vi "Advanced data viewer.vi"() -> ()   [LabVIEW 2016]
uses:
  <vilib>/Utility/miscctls.llb/LV3DPointTypeDef.ctl
  Typedef/Advancer viewer - States.ctl
  <vilib>/picture/3D Picture Control/Object/Create Object (name).vi
  <vilib>/picture/3D Picture Control/NI_3D Picture Control.lvlib
panel:
  out "Intensity Graph":sgl[][](graph)
  in  "Clear plot":bool
  out "Strain 1-8 Zoom":T1(graph)
  out "3D Picture":refnum<vi>(3d-picture)
  out "Strain 1-8":T1(graph)
  # "Yaw - Pitch - Roll - 3D"
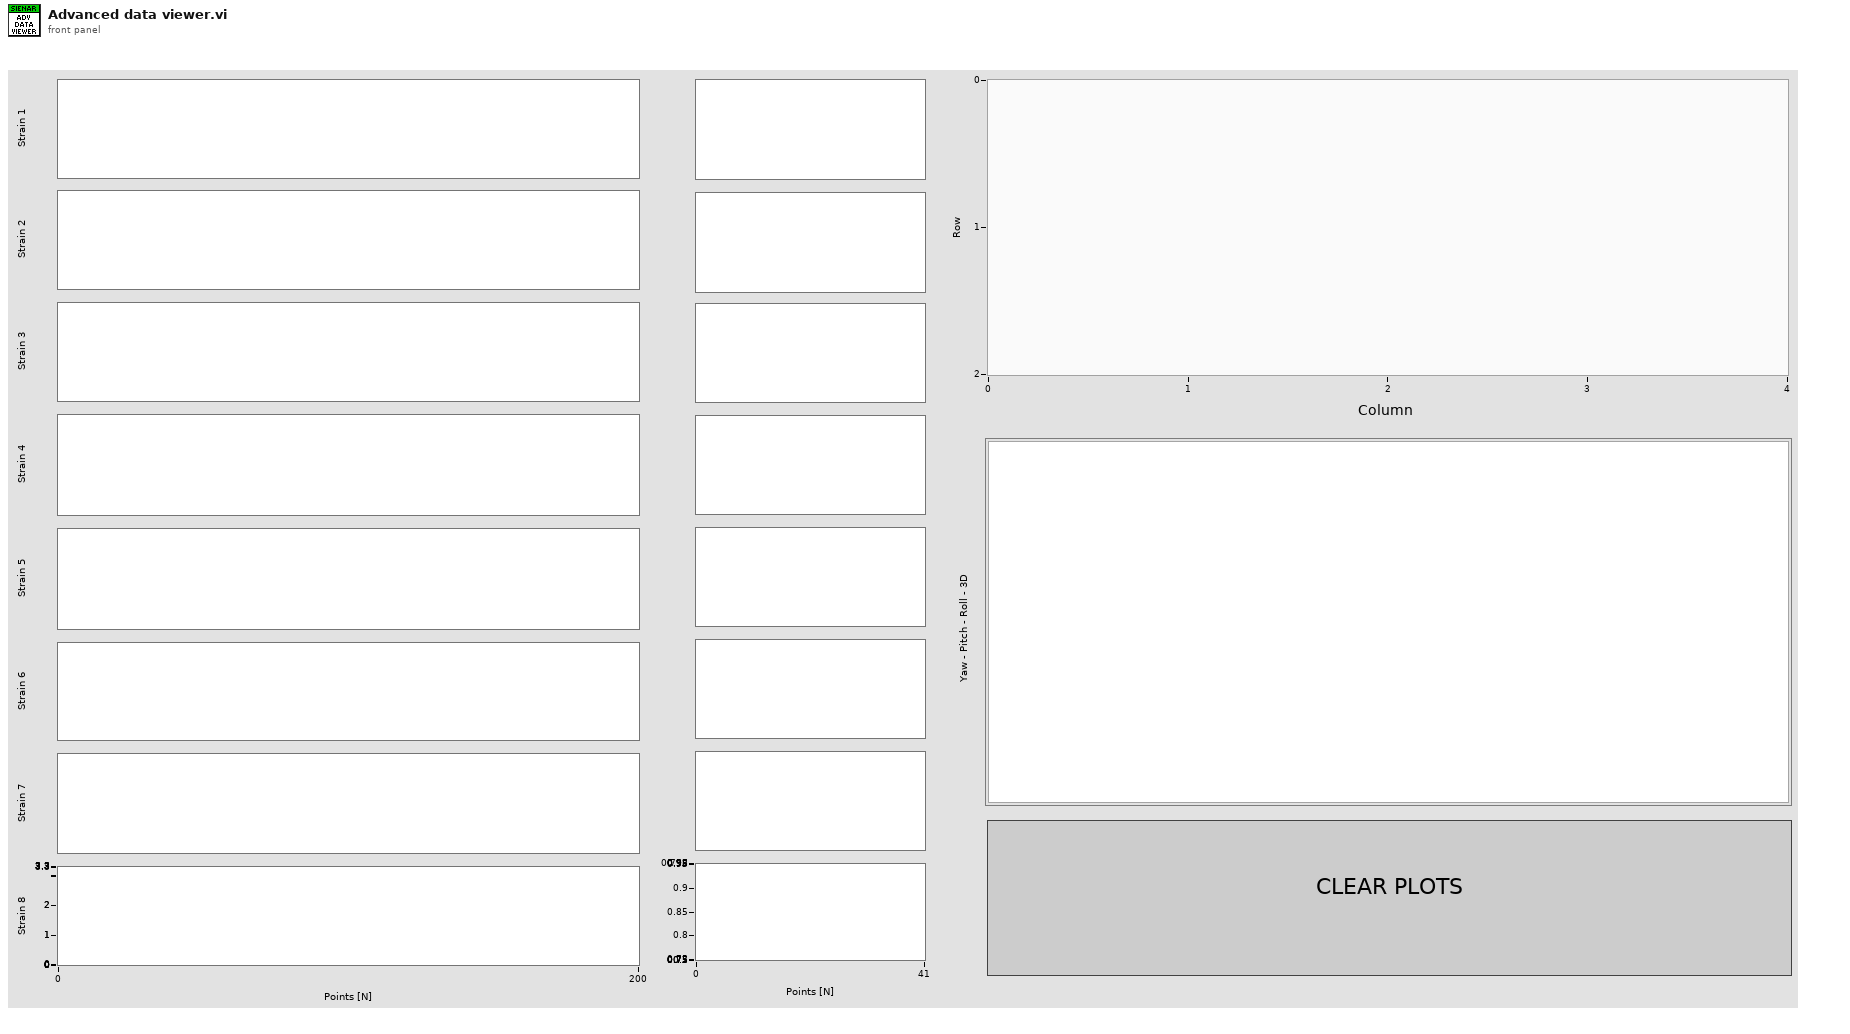
[diagram p1: front panel]
types:
  T1 = cluster{"Strain sensor 1":sgl, "Strain sensor 2":sgl, "Strain sensor 3":sgl, "Strain sensor 4":sgl, "Strain sensor 5":sgl, "Strain sensor 6":sgl, "Strain sensor 7":sgl, "Strain sensor 8":sgl}
  T2 = cluster{"Strain data":cluster{"Strain sensor 1":sgl, "Strain sensor 2":sgl, "Strain sensor 3":sgl, "Strain sensor 4":sgl, "Strain sensor 5":sgl, "Strain sensor 6":sgl, "Strain sensor 7":sgl, "Strain sensor 8":sgl}, "YPR data":cluster{"Yaw":sgl, "Pitch":sgl, "Roll":sgl}}
  T3 = typedef "Advancer viewer - States.ctl" = enum16{"Run data", "Exit"}
  T4 = typedef "LV3DPointTypeDef.ctl" = cluster{"X":sgl, "Y":sgl, "Z":sgl}
  T5 = cluster{"[0]":dbl, "[1]":dbl, "[2]":dbl, "[3]":dbl}[]
  T6 = cluster{"[0]":dbl, "[1]":dbl, "[2]":dbl, "[3]":dbl, "[4]":dbl, "[5]":dbl, "[6]":dbl, "[7]":dbl}[]
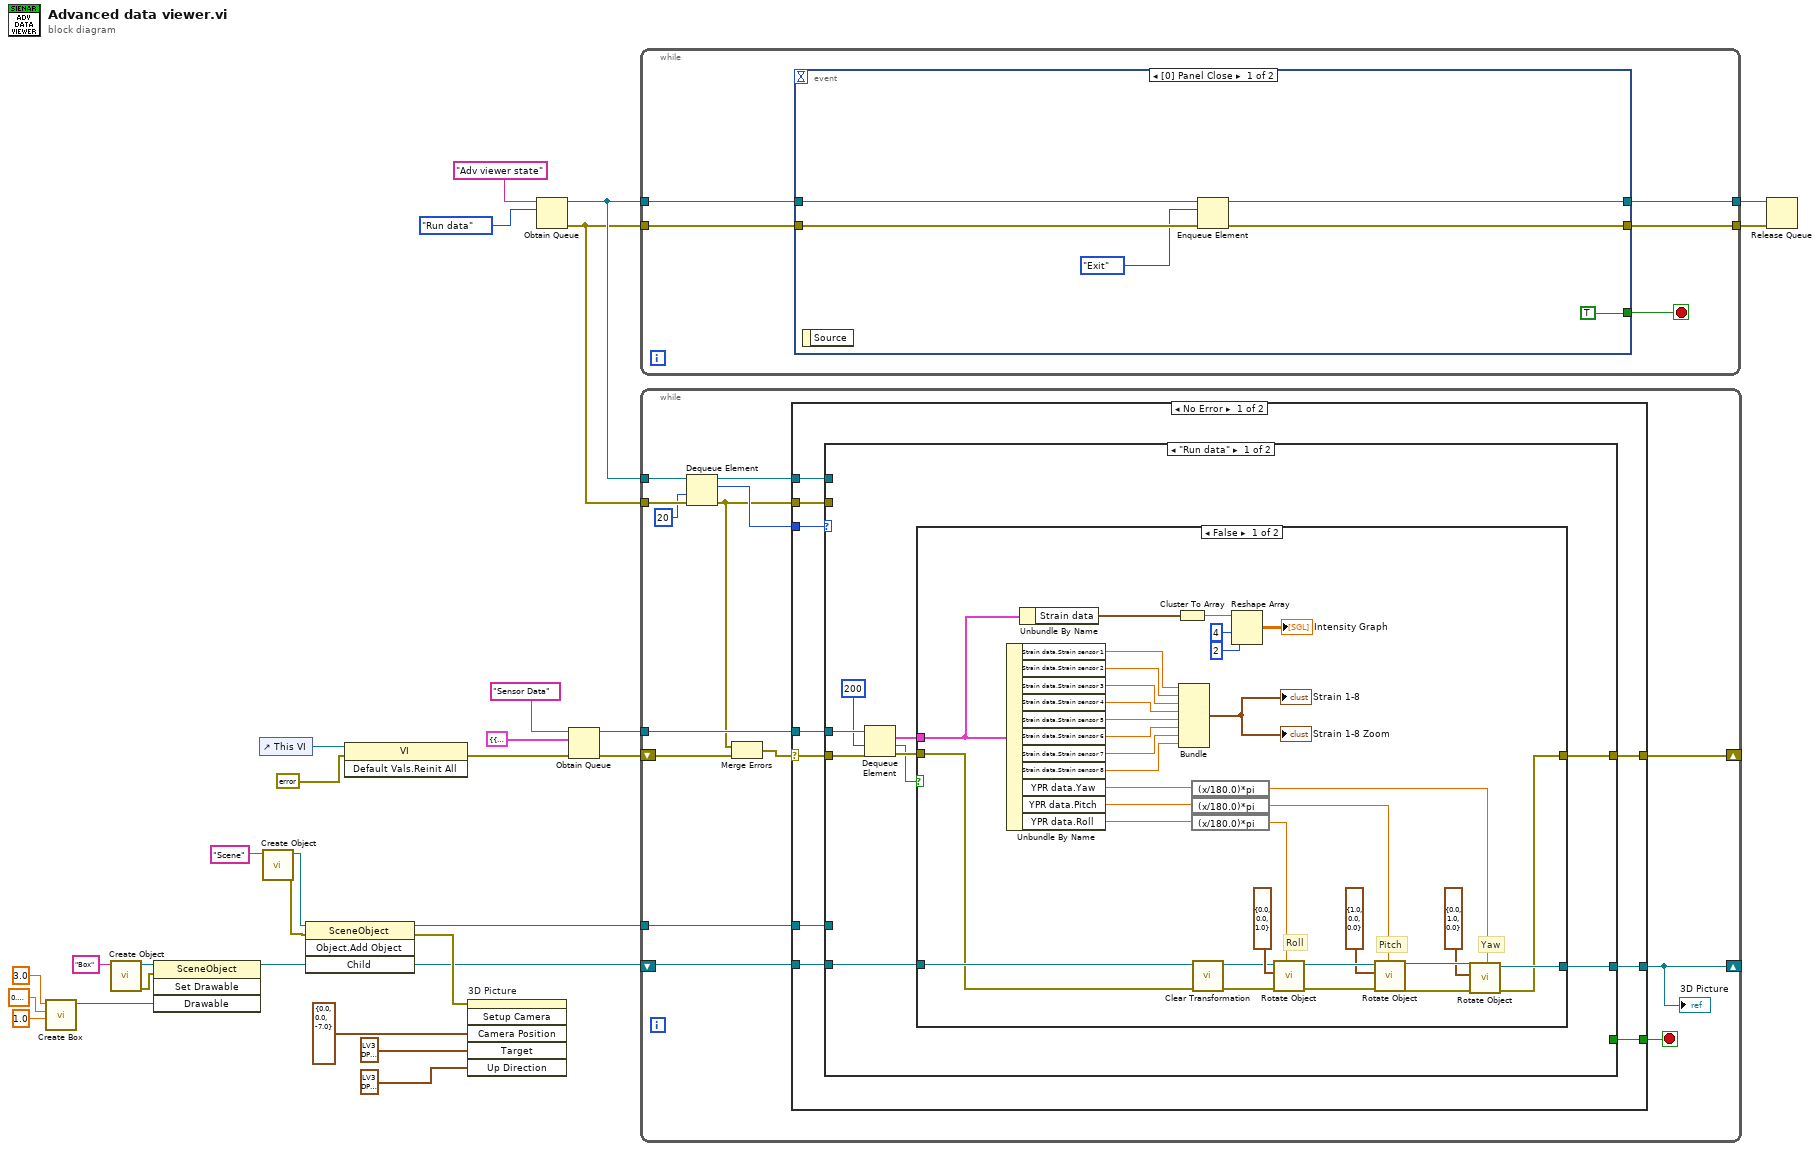
[diagram p0: block diagram]
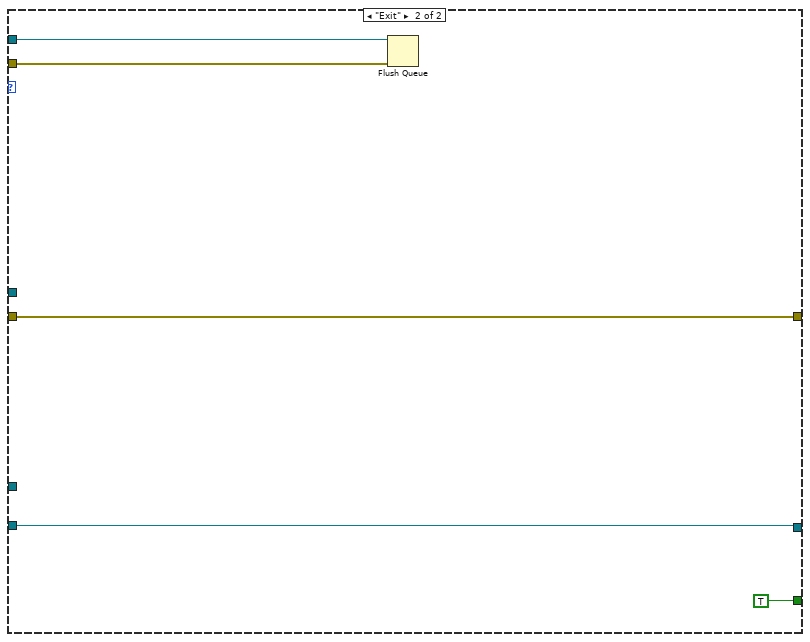
[diagram p3: hidden frame]
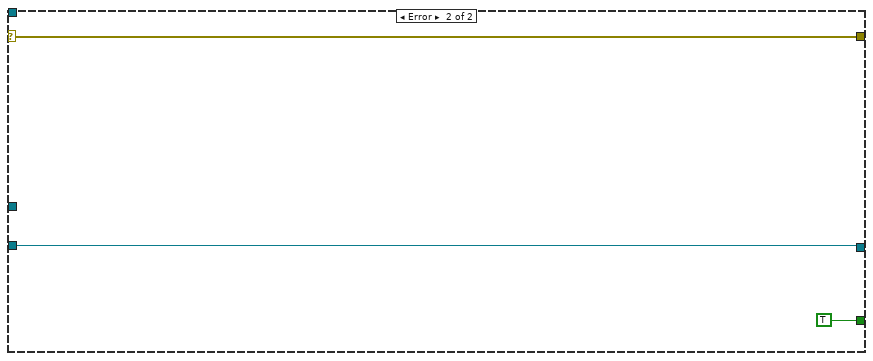
[diagram p4: hidden frame]
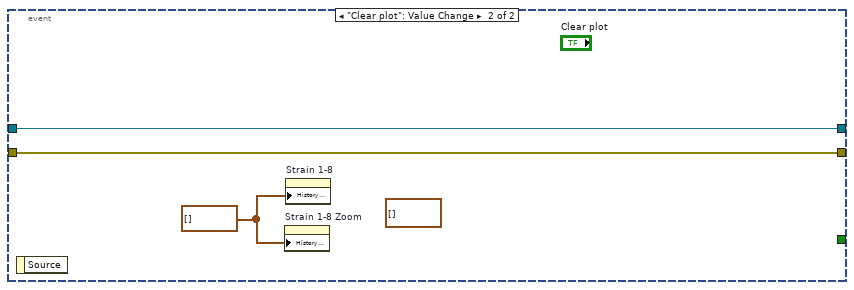
[diagram p5: hidden frame]
diagram:
  n1 = call <vilib>:"Create Box.vi"("Length Z"=sgl 1.0, "Length Y"=sgl 0.2, "Length X"=sgl 3.0) -> ("New Box Refnum"=w25:refnum<vi>)  [unwired: 7 in, 1 out]
  n2 = call-poly <vilib>:"Create Object.vi"("Name"="Box") -> ("error out"=w24:errorcluster, "Scene:New Object"=w23:refnum<vi>)  [unwired: 9 in]
  n3 = invoke class="SceneObject" method="Set Drawable"(reference=w23, error in=w24, "Drawable"=w25) -> (reference out=w29:refnum<vi>)  [unwired: 1 in, 3 out]
  n4 = control-ref of="This VI"() -> (w30:refnum<vi>)
  n5 = call-poly <vilib>:"Create Object.vi"("Name"="Scene") -> ("error out"=w28:errorcluster, "Scene:New Object"=w27:refnum<vi>)  [unwired: 9 in]
  n6 = invoke class="SceneObject" method="Object.Add Object"(reference=w27, error in=w28, "Child"=w29) -> (reference out=w5:refnum<vi>, error out=w15:errorcluster, "Child"=w6:refnum<vi>)  [unwired: 1 in, 1 out]
  n7 = invoke class="VI" method="Default Vals.Reinit All"(reference=w30, error in=errorcluster {"status"=FALSE, "code"=0, "source"=""} ("Error In")) -> (error out=w13:errorcluster)  [unwired: 1 in, 2 out]
  n8 = invoke on="3D Picture" class="SceneGraphDisp (strict)" method="Setup Camera"(error in=w15, "Camera Position"=T4 {"X"=0.0, "Y"=0.0, "Z"=-7.0}, "Target"=T4 {"X"=0.0, "Y"=0.0, "Z"=0.0}, "Up Direction"=T4 {"X"=0.0, "Y"=1.0, "Z"=0.0}) -> ()  [unwired: 2 in, 6 out]
  n9 = Obtain Queue(name (unnamed)="Adv viewer state", element data type=Advancer_viewer_-_States."Run data") -> (queue out=w11:refnum<queue>, error out=w10:errorcluster)  [unwired: 3 in, 1 out]
  n10 = Obtain Queue(name (unnamed)="Sensor Data", element data type=T2 {"Strain data"={"Strain sensor 1"=0.0, "Strain sensor 2"=0.0, "Strain sensor 3"=0.0, "Strain sensor 4"=0.0, "Strain sensor 5"=0.0, "Strain sensor 6"=0.0, "Strain sensor 7"=0.0, "Strain sensor 8"=0.0}, "YPR data"={"Yaw"=0.0, "Pitch"=0.0, "Roll"=0.0}} ("Wristband data"), error in (no error)=w13) -> (queue out=w8:refnum<queue>, error out=w7:errorcluster)  [unwired: 2 in, 1 out]
  n11 = while {
    tunnel: w11 -> [w34]
    tunnel: w10 -> [w33]
    tunnel: [w32] -> w3
    tunnel: [w31] -> w2
    stop <- w35 stop-if-true
    n12 = event shown="[0] Panel Close" {
      selector: _ -> [_ _]
      dyn-events: _ -> [_ _]
      timeout: _ -> [_ _]
      tunnel: [TRUE _] -> w35
      tunnel: w34 -> [w40 w42]
      tunnel: w33 -> [w39 w43]
      tunnel: [w38 w42] -> w32
      tunnel: [w37 w43] -> w31
      event Panel Close {
        n13 = event-data() -> ()  [unwired: 1 in, 1 out]
        n14 = Enqueue Element(queue=w40, element=Advancer_viewer_-_States."Exit", error in (no error)=w39) -> (queue out=w38:refnum<queue>, error out=w37:errorcluster)  [unwired: 1 in, 1 out]
      }
      event "Clear plot": Value Change {
        (unwired) T5 [] ("History Data")
        w44 = T6 [] ("History Data")
        n15 = event-data() -> ()  [unwired: 1 in, 1 out]
        n16 = property on="Strain 1-8 Zoom" class="WFChart (strict)"("History Data"=w44) -> ()  [unwired: 2 in, 2 out]
        n17 = property on="Strain 1-8" class="WFChart (strict)"("History Data"=w44) -> ()  [unwired: 2 in, 2 out]
      }
    }
  }
  n18 = while {
    tunnel: w11 -> [w58]
    tunnel: w10 -> [w57]
    tunnel: w8 -> [w55]
    tunnel: w5 -> [w53]
    shift-right: [w49] -> _
    shift-left: w6 -> [w54]
    shift-right: [w45] -> _
    shift-left: w7 -> [w48]
    stop <- w50 stop-if-true
    n19 = Dequeue Element(queue=w58, timeout in ms (-1)=20, error in (no error)=w57) -> (queue out=w52:refnum<queue>, element=w56:T3, error out=w46:errorcluster)  [unwired: 1 out]
    n20 = Merge Errors(w46, w48) -> (w47:errorcluster)
    n21 = case shown="No Error" w47 {
      selector: w47 -> [w60 w119]
      tunnel: w56 -> [w68 _]
      tunnel: w55 -> [w67 _]
      tunnel: w54 -> [w66 w120]
      tunnel: w53 -> [w65 _]
      tunnel: w52 -> [w64 _]
      tunnel: w46 -> [w63 _]
      tunnel: [w62 TRUE] -> w50
      tunnel: [w61 w120] -> w49
      tunnel: [w59 w119] -> w45
      frame No Error {
        n22 = case shown="\"Run data\"" w68 {
          tunnel: w67 -> [w77 _]
          tunnel: w60 -> [w76 w114]
          tunnel: w66 -> [w75 w115]
          tunnel: w65 -> [_ _]
          tunnel: w64 -> [_ w118]
          tunnel: w63 -> [_ w117]
          tunnel: [_ TRUE] -> w62
          tunnel: [w73 w115] -> w61
          tunnel: [w71 w114] -> w59
          frame "Run data" {
            n23 = Dequeue Element(queue=w77, timeout in ms (-1)=200, error in (no error)=w76) -> (element=w72:T2, timed out?=w70:bool, error out=w74:errorcluster)  [unwired: 1 out]
            n24 = case shown="False" w70 {
              tunnel: w75 -> [w100 w112]
              tunnel: w74 -> [w90 w113]
              tunnel: [w86 w112] -> w73
              tunnel: w72 -> [w85 _]
              tunnel: [w78 w113] -> w71
              frame False {
                # "Yaw"
                # "Pitch"
                # "Roll"
                n25 = Unbundle By Name(w85) -> ("Strain data.Strain sensor 1"=w108:sgl, "Strain data.Strain sensor 2"=w107:sgl, "Strain data.Strain sensor 3"=w106:sgl, "Strain data.Strain sensor 4"=w105:sgl, "Strain data.Strain sensor 5"=w104:sgl, "Strain data.Strain sensor 6"=w103:sgl, "Strain data.Strain sensor 7"=w102:sgl, "Strain data.Strain sensor 8"=w101:sgl, "YPR data.Yaw"=w81:sgl, "YPR data.Pitch"=w80:sgl, "YPR data.Roll"=w79:sgl)
                n26 = Unbundle By Name(w85) -> ("Strain data"=w84:T1)
                n27 = Cluster To Array(cluster=w84) -> (array=w109:sgl[])
                n28 = Bundle("Strain sensor 1"=w108, "Strain sensor 2"=w107, "Strain sensor 3"=w106, "Strain sensor 4"=w105, "Strain sensor 5"=w104, "Strain sensor 6"=w103, "Strain sensor 7"=w102, "Strain sensor 8"=w101) -> (→"Strain 1-8" →"Strain 1-8 Zoom":T1)  [unwired: 1 in]
                n29 = expression code="(x/180.0)*pi" ("degrees to radians")(w81) -> (w87:sgl)
                n30 = expression code="(x/180.0)*pi" ("degrees to radians")(w80) -> (w88:sgl)
                n31 = expression code="(x/180.0)*pi" ("degrees to radians")(w79) -> (w89:sgl)
                n32 = call <vilib>:"Clear Transformation.vi"("error in (no error)"=w90, "Object Refnum In"=w100) -> ("error out"=w91:errorcluster, "Object Refnum Out"=w92:refnum<vi>)  [unwired: 8 in]
                n33 = Reshape Array(w109, 4 ("dimension size"), 2 ("dimension size")) -> (→"Intensity Graph":sgl[][])
                n34 = call <vilib>:"Rotate Object.vi"("error in (no error)"=w91, "Angle"=w89, "Axis"=cluster{"X":sgl, "Y":sgl, "Z":sgl} {"X"=0.0, "Y"=0.0, "Z"=1.0}, "Scene.Object In"=w92) -> ("error out"=w98:errorcluster, "Scene.Object Out"=w99:refnum<vi>)  [unwired: 6 in]
                n35 = call <vilib>:"Rotate Object.vi"("error in (no error)"=w98, "Angle"=w88, "Axis"=cluster{"X":sgl, "Y":sgl, "Z":sgl} {"X"=1.0, "Y"=0.0, "Z"=0.0} ("Axis 2"), "Scene.Object In"=w99) -> ("error out"=w95:errorcluster, "Scene.Object Out"=w96:refnum<vi>)  [unwired: 6 in]
                n36 = call <vilib>:"Rotate Object.vi"("error in (no error)"=w95, "Angle"=w87, "Axis"=cluster{"X":sgl, "Y":sgl, "Z":sgl} {"X"=0.0, "Y"=1.0, "Z"=0.0} ("Axis 3"), "Scene.Object In"=w96) -> ("error out"=w78:errorcluster, "Scene.Object Out"=w86:refnum<vi>)  [unwired: 6 in]
              }
              frame True {
              }
            }
          }
          frame "Exit" {
            n37 = Flush Queue(queue=w118, error in (no error)=w117) -> ()  [unwired: 3 out]
          }
        }
      }
      frame Error {
      }
    }
    "3D Picture" <- w49
  }
  n38 = Release Queue(queue=w3, error in (no error)=w2) -> ()  [unwired: 1 in, 3 out]
